vi "Refresh FP Items.vi"(8 "error in (no error)":errorcluster, 10 "FP Item Props in":T1, 11 "Array in":refnum<vi>) -> (0 "error out":errorcluster)   [LabVIEW 2020, in "DocTool.lvlib"]
uses:
  DocTool.lvlib
  TDefs/FP Items Properties.ctl
  TDefs/FP Item Properties.ctl
  TDefs/CopyTag.ctl
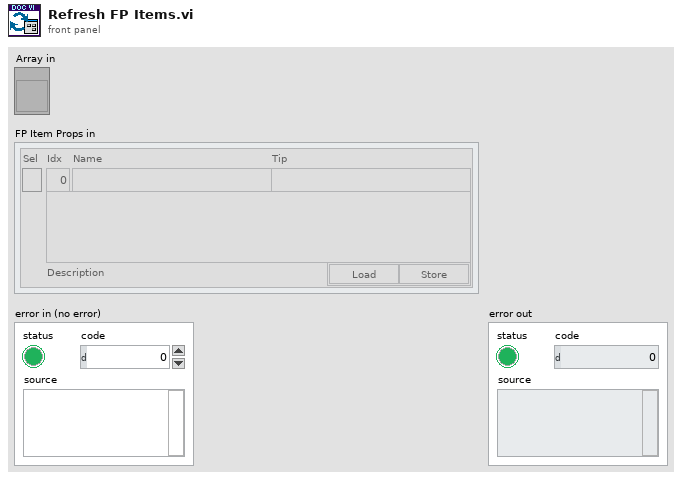
[diagram p1: front panel]
types:
  T1 = typedef "DocTool.lvlib/FP Items Properties.ctl" = T2[]
  T2 = typedef "DocTool.lvlib/FP Item Properties.ctl" = cluster{"Sel":bool, "Idx":i32, "Name":string, "Description":string, "Tip":string, "Load Store":T3}
  T3 = typedef "DocTool.lvlib/CopyTag.ctl" = cluster{"Load":bool, "Store":bool}
  T4 = enum8{"Enabled", "Disabled", "Disabled and Grayed Out"}
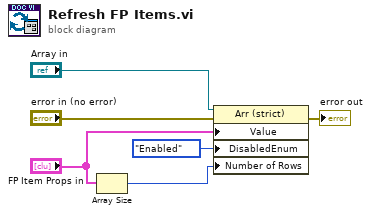
[diagram p0: block diagram]
diagram:
  n1 = Array Size(array="FP Item Props in") -> (size(s)=w1:i32)
  n2 = property class="Arr (strict)"(reference="Array in", error in="error in (no error)", "Value"="FP Item Props in", "DisabledEnum"=T4."Enabled" ("Disabled"), "Number of Rows"=w1) -> (error out=→"error out":errorcluster)  [unwired: 1 out]
